vi "File List Remove and next.vi"(11 "File List in":refnum<class "File List.lvclass">) -> (1 "Current file index out":i32, 2 "Current file out":path, 3 "File List out":refnum<class "File List.lvclass">)   [LabVIEW 2014, in "COSYLib.lvlib" / "File List.lvclass"]
doc: "Removes the current file, and activates and returns the next one in the list.\nIf there are no remaining files to be activated, an empty path and -1 are returned."
uses:
  File List.lvclass
  File List.lvclass/File List.ctl
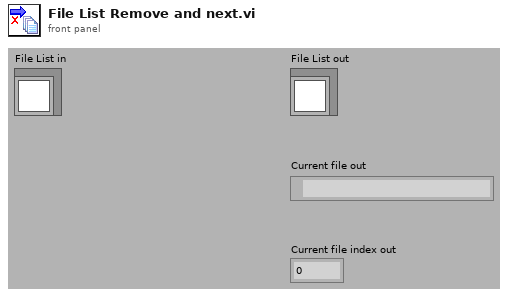
[diagram p1: front panel]
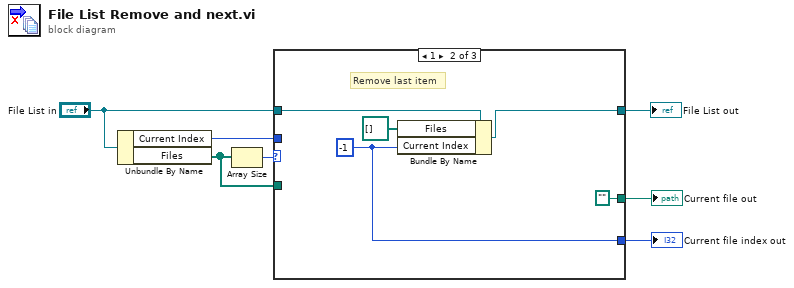
[diagram p0: block diagram]
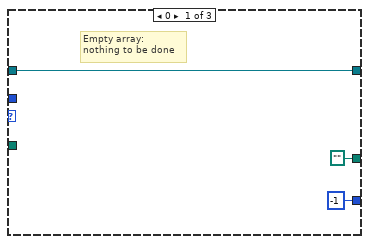
[diagram p2: hidden frame]
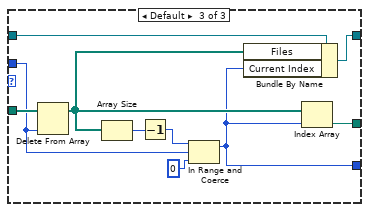
[diagram p3: hidden frame]
diagram:
  n1 = Unbundle By Name("File List in") -> ("Current Index"=w6:i32, "Files"=w1:path[])
  n2 = Array Size(array=w1) -> (size(s)=w7:i32)
  n3 = case shown="1" w7 {
    tunnel: w6 -> [_ _ w21]
    tunnel: [path "" path "" w17] -> w5
    tunnel: [-1 w12 w16] -> w4
    tunnel: "File List in" -> [w8 w15 w20]
    tunnel: [w8 w14 w19] -> w2
    tunnel: w1 -> [_ _ w25]
    frame 0 {
      # "Empty array:\nnothing to be done"
    }
    frame 1 {
      w12 = -1 ("Current Index")
      # "Remove last item"
      n4 = Bundle By Name(cluster=w15, "Files"=path[] [], "Current Index"=w12) -> (w14:refnum<class "File List.lvclass">)
    }
    frame Default {
      n5 = Delete From Array(array=w25, index=w21) -> (array with subset deleted=w18:path[])  [unwired: 1 in, 1 out]
      n6 = Array Size(array=w18) -> (size(s)=w24:i32)
      n7 = Decrement(x=w24) -> (x-1=w23:i32)
      n8 = In Range and Coerce(upper limit=w23, x=w21, lower limit=0) -> (coerced(x)=w16:i32)  [unwired: 1 out]
      n9 = Bundle By Name(cluster=w20, "Files"=w18, "Current Index"=w16) -> (w19:refnum<class "File List.lvclass">)
      n10 = Index Array(array=w18, index=w16) -> (element=w17:path)
    }
  }
  "File List out" <- w2
  "Current file out" <- w5
  "Current file index out" <- w4
